vi "State to Status String.vi"(11 "State":T1) -> (3 "Status String":string)   [LabVIEW 2014]
uses:
  Scripting/Scripting States.ctl
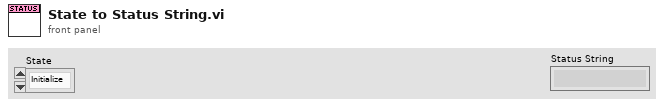
[diagram p1: front panel]
types:
  T1 = typedef "Scripting States.ctl" = enum16{"Initialize", "Modify Dequeue Commands", "Modify Enqueue Data", "Create Project FIFOs", "Create and Place IO Nodes", "Update Node Count in Engine", "Expand FIFO Type Def", "Populate FIFO Names in Engine", "Modify I/O Pin Names", "Modify I/O Pin Enable", "Replace DLU", "Place SPI Engine", "Buses Complete Check", "End"}
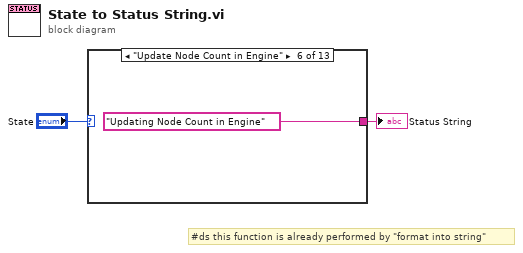
[diagram p0: block diagram]
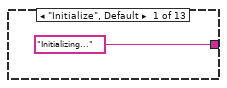
[diagram p2: hidden frame]
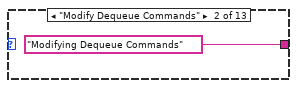
[diagram p3: hidden frame]
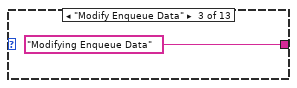
[diagram p4: hidden frame]
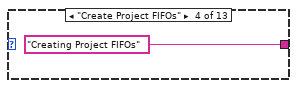
[diagram p5: hidden frame]
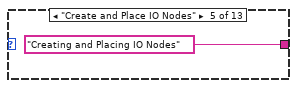
[diagram p6: hidden frame]
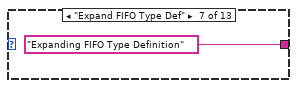
[diagram p7: hidden frame]
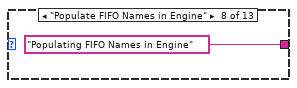
[diagram p8: hidden frame]
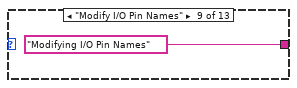
[diagram p9: hidden frame]
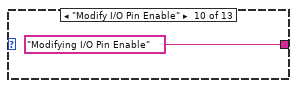
[diagram p10: hidden frame]
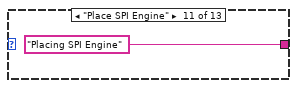
[diagram p11: hidden frame]
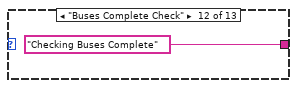
[diagram p12: hidden frame]
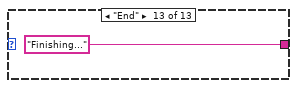
[diagram p13: hidden frame]
diagram:
  # "#ds this function is already performed by \"format into string\""
  n1 = case shown="\"Update Node Count in Engine\"" "State" {
    tunnel: ["Initializing..." "Modifying Dequeue Commands" "Modifying Enqueue Data" "Creating Project FIFOs" "Creating and Placing IO Nodes" "Updating Node Count in Engine" "Expanding FIFO Type Definition" "Populating FIFO Names in Engine" "Modifying I/O Pin Names" "Modifying I/O Pin Enable" "Placing SPI Engine" "Checking Buses Complete" "Finishing..."] -> w1
    frame "Initialize", Default {
    }
    frame "Modify Dequeue Commands" {
    }
    frame "Modify Enqueue Data" {
    }
    frame "Create Project FIFOs" {
    }
    frame "Create and Place IO Nodes" {
    }
    frame "Update Node Count in Engine" {
    }
    frame "Expand FIFO Type Def" {
    }
    frame "Populate FIFO Names in Engine" {
    }
    frame "Modify I/O Pin Names" {
    }
    frame "Modify I/O Pin Enable" {
    }
    frame "Place SPI Engine" {
    }
    frame "Buses Complete Check" {
    }
    frame "End" {
    }
  }
  "Status String" <- w1
